vi "Write async.vi"(8 "error in":errorcluster, 10 "async module":refnum<class "asynchronous execution module configuration.lvclass">, 11 "module editor node in":refnum<class "module editor node.lvclass">) -> (0 "error out":errorcluster, 3 "module editor node out":refnum<class "module editor node.lvclass">)   [LabVIEW 2013, in "PL Framework Configuration Tool.lvlib" / "module editor node.lvclass"]
uses:
  module editor node.lvclass
  asynchronous execution module/configuration/asynchronous execution module configuration.lvclass
  module editor node.lvclass/module editor node.ctl
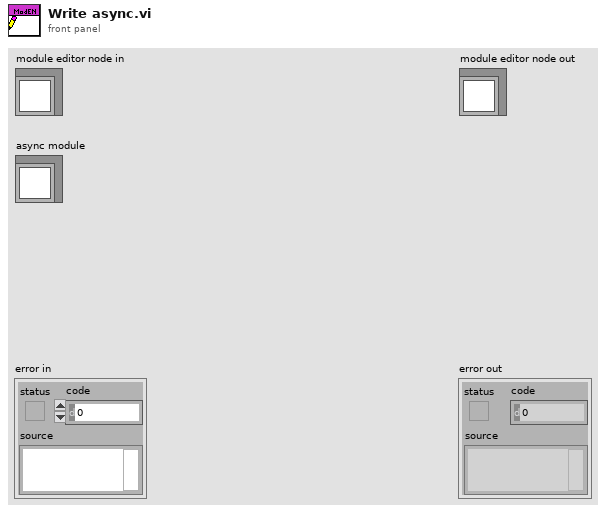
[diagram p1: front panel]
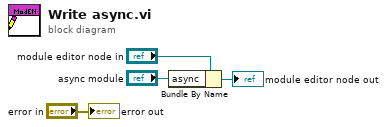
[diagram p0: block diagram]
diagram:
  n1 = Bundle By Name(cluster="module editor node in", "async"="async module") -> (→"module editor node out":refnum<class "module editor node.lvclass">)
  "error out" <- "error in"
